vi "timestring_4.vi"(8 "error in (no error)":errorcluster, 10 "String Array In":string[](array[string])) -> (0 "error out":errorcluster, 2 "Time Stamp Out":timestamp[](array[timestamp]) format="%<%X>T")   [LabVIEW 2017]
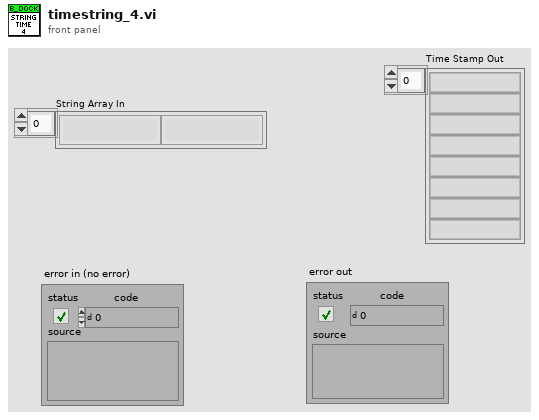
[diagram p1: front panel]
types:
  T1 = cluster{"second":i32, "minute":i32, "hour":i32, "day of month":i32, "month":i32, "year":i32, "day of week":i32, "day of year":i32, "is DST":i32}
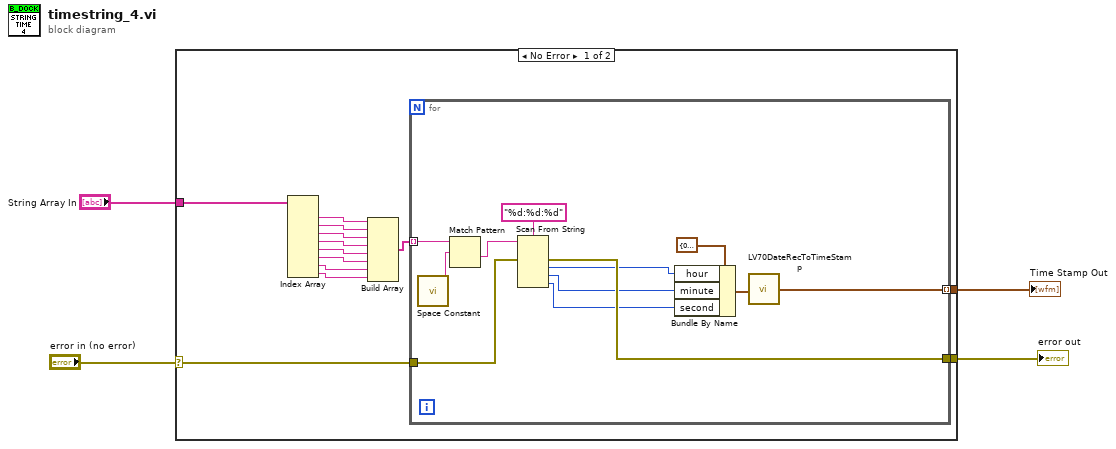
[diagram p0: block diagram]
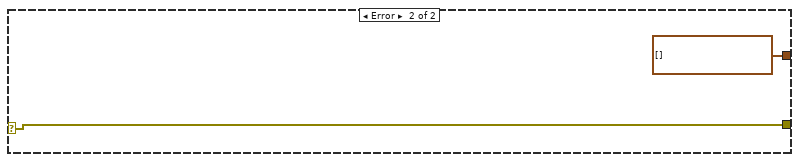
[diagram p2: hidden frame]
diagram:
  n1 = case shown="No Error" "error in (no error)" {
    selector: "error in (no error)" -> [w10 w31]
    tunnel: "String Array In" -> [w17 _]
    tunnel: [w12 timestamp[] []] -> w3
    tunnel: [w9 w31] -> w1
    frame No Error {
      n2 = Index Array(array=w17) -> (element #1=w7:string, element #2=w16:string, element #3=w15:string, element #4=w14:string, element #5=w13:string, element #6=w11:string, element #7=w6:string, element #8=w5:string)  [unwired: 8 in]
      n3 = Build Array(w7, w16, w15, w14, w13, w11, w6, w5) -> (w8:string[])
      n4 = for {
        tunnel: w8 -> [w24] mode=indexing
        tunnel: [w28] -> w12 mode=indexing
        tunnel: w10 -> [w27]
        tunnel: [w26] -> w9
        n5 = call <vilib>:"Space Constant.vi"() -> ("String"=w25:string)
        n6 = Match Pattern(string=w24, regular expression=w25) -> (after substring=w23:string)  [unwired: 1 in, 3 out]
        n7 = Scan From String(format string="%d:%d:%d", input string=w23, error in=w27) -> (error out=w26:errorcluster, output 1=w20:i32, output 2=w19:i32, output 3=w18:i32)  [unwired: 4 in, 2 out]
        n8 = Bundle By Name(cluster=T1 {"second"=0, "minute"=0, "hour"=0, "day of month"=1, "month"=1, "year"=2018, "day of week"=0, "day of year"=0, "is DST"=0} ("date time rec"), "hour"=w20, "minute"=w19, "second"=w18) -> (w22:T1)
        n9 = call <vilib>:"LV70DateRecToTimeStamp.vi"("date time rec"=w22) -> ("Time Stamp"=w28:timestamp)
      }
    }
    frame Error {
    }
  }
  "Time Stamp Out" <- w3
  "error out" <- w1
